vi "PUSH_ASR_COUNT.vi"(8 "error in (no error)":errorcluster, 11 "Ref In":T1={"MS SQL Connection"=refnum, "UDL File"=path "", "Time"="", "DCODE"="", "WIP+1"=0, "MC No?"=0, "POKAYOKE?"=FALSE, "Expected Result"="", "Result [Status]"="", "Clock"=0.0, "RFID"="", "WIP Queue"=refnum, "TS Parameter"={"ProfitCenterCode"="", "LineCode"="", "WorkOrderNumber"="", "Model"="", "Model_with_Prefix"="", "VendorCode"="", "SetParameterDateCode"="", "PokaYoke"=0, "Target"=1, "Live_DateCode"="", "CustomerPartNumber"="", "Hand"="", "sBarcode"=FALSE, "FCA"=0, "Ent_Stamp"=timestamp(0 s since 1904-01-01), "STS_CD"=0.0}, "Data_Queue"=[], "RFID Serial No."=""} {"TS Parameter"."FCA" format="%01d"; "TS Parameter"."Target" min=1 max=100000; "TS Parameter"."PokaYoke" min=0 max=1}) -> (0 "error out":errorcluster, 1 "PASS":i32, 2 "FAIL":i32, 3 "Ref Out":T1={"MS SQL Connection"=refnum, "UDL File"=path "", "Time"="", "DCODE"="", "WIP+1"=0, "MC No?"=0, "POKAYOKE?"=FALSE, "Expected Result"="", "Result [Status]"="", "Clock"=0.0, "RFID"="", "WIP Queue"=refnum, "TS Parameter"={"ProfitCenterCode"="", "LineCode"="", "WorkOrderNumber"="", "Model"="", "Model_with_Prefix"="", "VendorCode"="", "SetParameterDateCode"="", "PokaYoke"=0, "Target"=1, "Live_DateCode"="", "CustomerPartNumber"="", "Hand"="", "sBarcode"=FALSE, "FCA"=0, "Ent_Stamp"=timestamp(0 s since 1904-01-01), "STS_CD"=0.0}, "Data_Queue"=[], "RFID Serial No."=""} {"TS Parameter"."FCA" format="%01d"; "TS Parameter"."Target" min=1 max=100000; "TS Parameter"."PokaYoke" min=0 max=1}, 5 "resulting string":string)   [LabVIEW 2020]
uses:
  Controls/TD SQL.ctl
  <vilib>/addons/database/Connection.llb/Conn ObjectReference.ctl
  Controls/WIP_State.ctl
  Controls/TS_Parameter.ctl
  <vilib>/addons/database/Connection.llb/Conn Execute.vi
  <vilib>/addons/database/Recordset.llb/Rec Fetch Recordset Data (R).vi
  <vilib>/addons/database/Recordset.llb/Rec Destroy - Connection.vi
  <vilib>/addons/database/NI_Database_API.lvlib
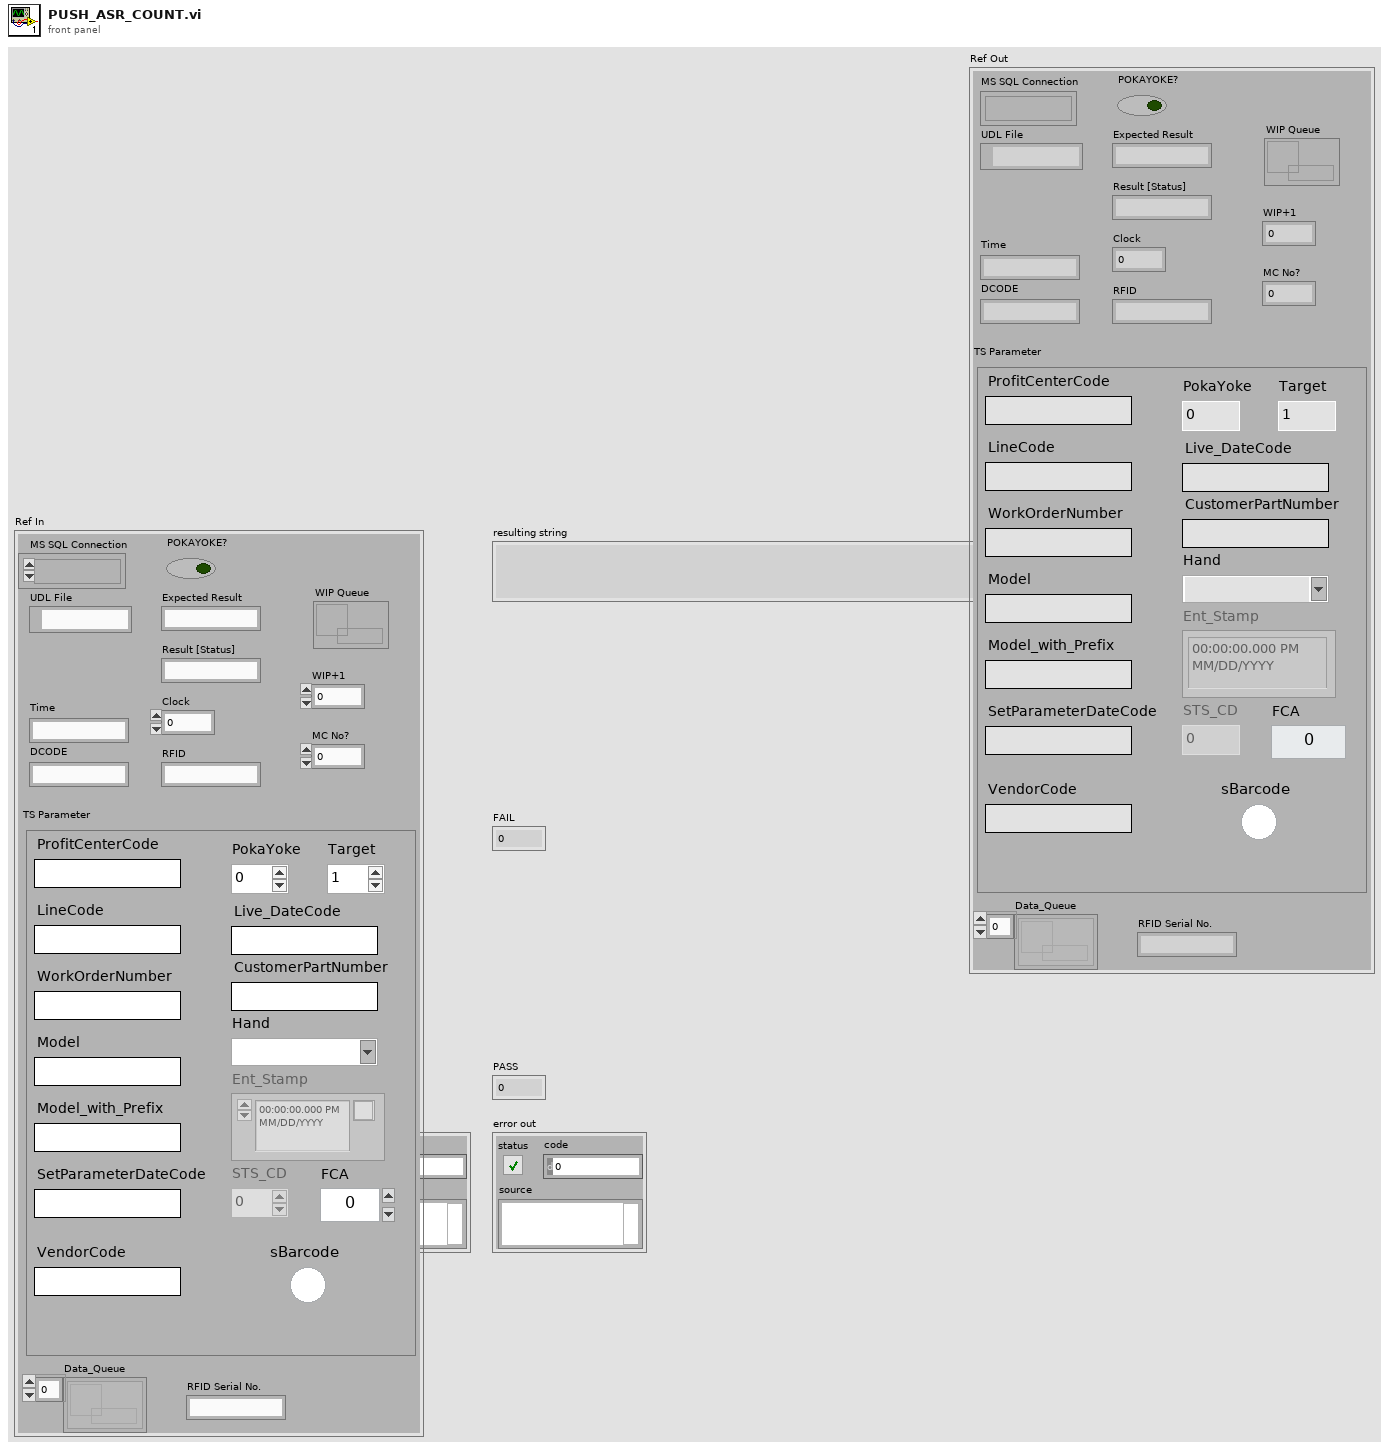
[diagram p1: front panel]
types:
  T1 = typedef "TD SQL.ctl" = cluster{"MS SQL Connection":T2, "UDL File":path, "Time":string, "DCODE":string, "WIP+1":i64, "MC No?":i32, "POKAYOKE?":bool, "Expected Result":string, "Result [Status]":string, "Clock":dbl, "RFID":string, "WIP Queue":refnum<queue>, "TS Parameter":T3, "Data_Queue":refnum<queue>[], "RFID Serial No.":string}
  T2 = typedef "NI_Database_API.lvlib/Conn ObjectReference.ctl" = refnum<k1>
  T3 = typedef "TS_Parameter.ctl" = cluster{"ProfitCenterCode":string, "LineCode":string, "WorkOrderNumber":string, "Model":string, "Model_with_Prefix":string, "VendorCode":string, "SetParameterDateCode":string, "PokaYoke":i32, "Target":i32, "Live_DateCode":string, "CustomerPartNumber":string, "Hand":string, "sBarcode":bool, "FCA":i32, "Ent_Stamp":timestamp, "STS_CD":dbl}
  T4 = typedef "NI_Database_API.lvlib/Rec ObjectReference.ctl" = refnum<k1>
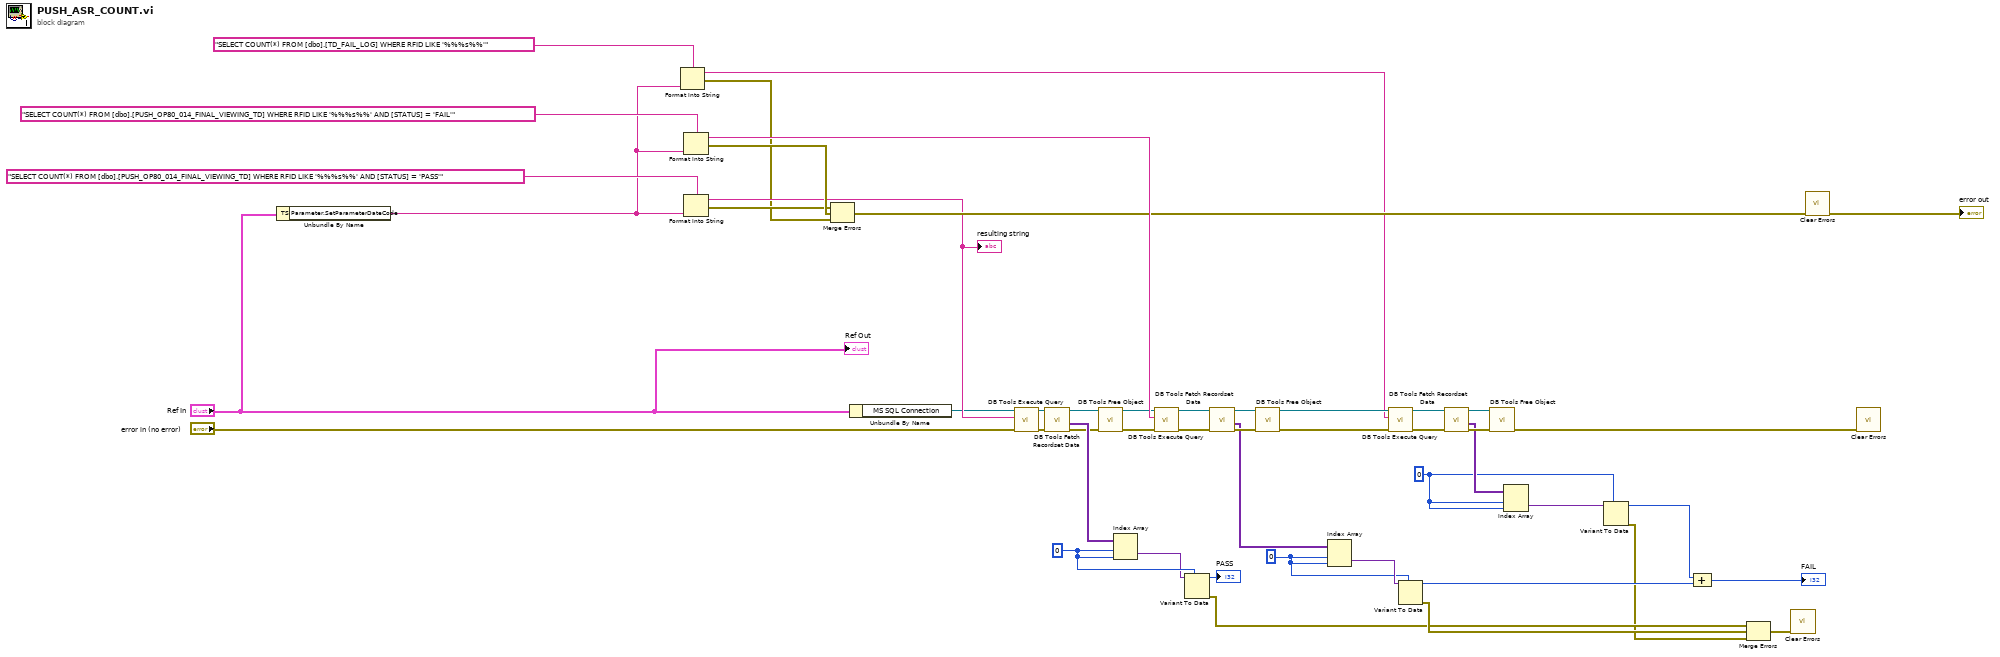
[diagram p0: block diagram]
diagram:
  w6 = 0 ("index (row)")
  w44 = 0 ("index (row)")
  w41 = 0 ("index (row)")
  n1 = Unbundle By Name("Ref In") -> ("TS Parameter.SetParameterDateCode"=w1:string)
  n2 = Format Into String(format string="SELECT COUNT(*) FROM [dbo].[TD_FAIL_LOG] WHERE RFID LIKE '%%%s%%'" ("Query"), w1) -> (resulting string=w11:string, error out=w17:errorcluster)  [unwired: 2 in]
  n3 = Format Into String(format string="SELECT COUNT(*) FROM [dbo].[PUSH_OP80_014_FINAL_VIEWING_TD] WHERE RFID LIKE '%%%s%%' AND [STATUS] = 'FAIL'" ("Query"), w1) -> (resulting string=w38:string, error out=w29:errorcluster)  [unwired: 2 in]
  n4 = Format Into String(format string="SELECT COUNT(*) FROM [dbo].[PUSH_OP80_014_FINAL_VIEWING_TD] WHERE RFID LIKE '%%%s%%' AND [STATUS] = 'PASS'" ("Query"), w1) -> (resulting string=w24:string, error out=w22:errorcluster)  [unwired: 2 in]
  "resulting string" <- w24
  n5 = Merge Errors(w22, w29, w17) -> (w28:errorcluster)
  n6 = Unbundle By Name("Ref In") -> ("MS SQL Connection"=w23:T2)
  n7 = call-poly <vilib>:"DB Tools Execute Query.vi"("error in (no error)"="error in (no error)", "SQL query"=w24, "connection reference"=w23) -> ("error out"=w26:errorcluster, "recordset reference"=w25:T4)  [unwired: 5 in]
  n8 = call-poly <vilib>:"DB Tools Fetch Recordset Data.vi"("error in (no error)"=w26, "recordset reference"=w25) -> ("error out"=w32:errorcluster, "recordset data"=w39:variant[][], "recordset reference out"=w33:T4)  [unwired: 3 in]
  n9 = call-poly <vilib>:"DB Tools Free Object.vi"("error in (no error)"=w32, "recordset reference"=w33) -> ("error out"=w35:errorcluster, "connection reference"=w34:T2)  [unwired: 8 in]
  n10 = Index Array(array=w39, index (row)=w41, index (col)=w41) -> (element=w40:variant)
  n11 = call-poly <vilib>:"DB Tools Execute Query.vi"("error in (no error)"=w35, "SQL query"=w38, "connection reference"=w34) -> ("error out"=w30:errorcluster, "recordset reference"=w31:T4)  [unwired: 5 in]
  n12 = Variant To Data(type=w41, Variant=w40) -> (data=→"PASS":i32, error out=w46:errorcluster)  [unwired: 1 in]
  n13 = call-poly <vilib>:"DB Tools Fetch Recordset Data.vi"("error in (no error)"=w30, "recordset reference"=w31) -> ("error out"=w37:errorcluster, "recordset data"=w20:variant[][], "recordset reference out"=w36:T4)  [unwired: 3 in]
  n14 = call-poly <vilib>:"DB Tools Free Object.vi"("error in (no error)"=w37, "recordset reference"=w36) -> ("error out"=w10:errorcluster, "connection reference"=w12:T2)  [unwired: 8 in]
  n15 = Index Array(array=w20, index (row)=w44, index (col)=w44) -> (element=w45:variant)
  n16 = call-poly <vilib>:"DB Tools Execute Query.vi"("error in (no error)"=w10, "SQL query"=w11, "connection reference"=w12) -> ("error out"=w16:errorcluster, "recordset reference"=w15:T4)  [unwired: 5 in]
  n17 = Variant To Data(type=w44, Variant=w45) -> (data=w43:i32, error out=w47:errorcluster)  [unwired: 1 in]
  n18 = call-poly <vilib>:"DB Tools Fetch Recordset Data.vi"("error in (no error)"=w16, "recordset reference"=w15) -> ("error out"=w13:errorcluster, "recordset data"=w8:variant[][], "recordset reference out"=w14:T4)  [unwired: 3 in]
  n19 = call-poly <vilib>:"DB Tools Free Object.vi"("error in (no error)"=w13, "recordset reference"=w14) -> ("error out"=w9:errorcluster)  [unwired: 8 in, 1 out]
  n20 = Index Array(array=w8, index (row)=w6, index (col)=w6) -> (element=w7:variant)
  n21 = Variant To Data(type=w6, Variant=w7) -> (data=w3:i32, error out=w5:errorcluster)  [unwired: 1 in]
  n22 = Compound Arithmetic op=ADD(w3, w43) -> (→"FAIL":i32)
  n23 = Merge Errors(w46, w47, w5) -> (w48:errorcluster)
  n24 = call <vilib>:"Clear Errors.vi"("error in (no error)"=w48) -> ()  [unwired: 5 in, 2 out]
  n25 = call <vilib>:"Clear Errors.vi"("error in (no error)"=w28) -> ("error out"=→"error out":errorcluster)  [unwired: 5 in, 1 out]
  n26 = call <vilib>:"Clear Errors.vi"("error in (no error)"=w9) -> ()  [unwired: 5 in, 2 out]
  "Ref Out" <- "Ref In"
